vi "HFRR ADV v015 new software.vi"() -> ()   [LabVIEW 2025] (continued)
        n324 = event-data() -> ()  [unwired: 1 in, 6 out]
        n325 = Unbundle By Name("Password 3") -> ("Service Password"=w414:string)
        n326 = call <vilib>:"Trim Whitespace.vi"("string"=w414) -> ("trimmed string"=w412:string)  [unwired: 1 in]
        n327 = Equal?(x=w412, y="Service@123") -> (x = y?=w413:bool)
        n328 = case shown="False" w413 {
          selector: w413 -> [w418 w420]
          frame False {
            n329 = local write "Service Password enable"(w418) -> ()
            n330 = property on="Service Password Log" class="Str"("Visible"=TRUE) -> ()  [unwired: 2 in, 2 out]
            n331 = property on="Tab Control 5" class="TabCtl (strict)"("Tabs Visible?"=TRUE ("Page Labels Display Visible?")) -> ()  [unwired: 2 in, 2 out]
          }
          frame True {
            n332 = property on="Service Password Log" class="Str"("Visible"=FALSE) -> ()  [unwired: 2 in, 2 out]
            "Service Password enable" <- w420
          }
        }
      }
      event "Sign In": Value Change {
        w422 = FALSE ("Visible")
        n333 = event-data() -> ()  [unwired: 1 in, 6 out]
        n334 = property on="About" class="Clust (strict)"("Visible"=w422) -> ()  [unwired: 2 in, 2 out]
        n335 = property on="Password 3" class="Clust (strict)"("Visible"=w422) -> ()  [unwired: 2 in, 2 out]
        n336 = property on="Service Password Log" class="Str"("Visible"=FALSE) -> ()  [unwired: 2 in, 2 out]
      }
      event "Info": Value Change {
        n337 = event-data() -> ()  [unwired: 1 in, 6 out]
        n338 = local read "Info"() -> (w424:bool)
        n339 = case shown="False" w424 {
          frame False {
            n340 = property on="About" class="Clust (strict)"("Visible"=FALSE) -> ()  [unwired: 2 in, 2 out]
          }
          frame True {
            n341 = property on="About" class="Clust (strict)"("Visible"=TRUE) -> ()  [unwired: 2 in, 2 out]
          }
        }
      }
      event "Calibration": Value Change {
        n342 = event-data() -> ()  [unwired: 1 in, 6 out]
        n343 = local read "Calibration"() -> (w428:bool)
        n344 = case shown="False" w428 {
          frame False {
            n345 = property on="Calibration 2" class="TabCtl (strict)"("Visible"=FALSE) -> ()  [unwired: 2 in, 2 out]
            n346 = local write "Cal Password"("" ("Cal Password")) -> ()
          }
          frame True {
            n347 = property on="Calibration 2" class="TabCtl (strict)"("Visible"=TRUE) -> ()  [unwired: 2 in, 2 out]
            n348 = local write "Cal Password"("" ("Cal Password")) -> ()
          }
        }
        n349 = property on="Wrong Password" class="Str"("Visible"=FALSE) -> ()  [unwired: 2 in, 2 out]
      }
      event "Cal Password": Value Change {
        n350 = event-data() -> ()  [unwired: 1 in, 6 out]
        n351 = local read "Cal Password"() -> (w436:string)
        n352 = call <vilib>:"Trim Whitespace.vi"("string"=w436) -> ("trimmed string"=w435:string)  [unwired: 1 in]
        n353 = Equal?(x=w435, y="Cal@321") -> (x = y?=w433:bool)
        n354 = case shown="True" w433 {
          frame False {
            n355 = property on="Wrong Password" class="Str"("Visible"=TRUE) -> ()  [unwired: 2 in, 2 out]
          }
          frame True {
            n356 = property on="Wrong Password" class="Str"("Visible"=FALSE) -> ()  [unwired: 2 in, 2 out]
            n357 = local write "Main Tab"(T2."About" ("Main Tab")) -> ()
            n358 = local write "Cal Password"("" ("Cal Password")) -> ()
            n359 = local write "Main Dashboard Buttons"(T1."About" ("Main Dashboard Buttons")) -> ()
            n360 = local write "Tab Control 5"(T12."Temperature Calibration" ("Tab Control 5")) -> ()
            n361 = property on="Calibration 2" class="TabCtl (strict)"("Visible"=FALSE) -> ()  [unwired: 2 in, 2 out]
            n362 = property on="Tab Control 5" class="TabCtl (strict)"("Tabs Visible?"=FALSE ("Page Labels Display Visible?")) -> ()  [unwired: 2 in, 2 out]
            n363 = local write "Calibration"(FALSE ("Calibration")) -> ()
          }
        }
      }
      event "Calibration Selection": Value Change {
        n364 = event-data() -> ()  [unwired: 1 in, 6 out]
        n365 = local read "Calibration Selection"() -> (w447:T8)
        n366 = case shown="\"Stroke Calibration\"" w447 {
          tunnel: [T7."Stroke" ("Main Calibration Tab") T7."Friction" ("Main Calibration Tab") T7."Main" ("Main Calibration Tab") T7."Temperature" ("Main Calibration Tab")] -> w446
          frame "Stroke Calibration" {
          }
          frame "Friction Force Calibration" {
          }
          frame Default {
          }
          frame "Temperature Calibration" {
          }
        }
        n367 = local write "Main Calibration Tab"(w446) -> ()
      }
      event "Back Stroke": Value Change {
        n368 = event-data() -> ()  [unwired: 1 in, 6 out]
        n369 = local write "Main Stroke Tab"(T9."Step 1" ("Main Stroke Tab")) -> ()
        n370 = local write "Main Calibration Tab"(T7."Main" ("Main Calibration Tab")) -> ()
        n371 = local write "Back Stroke"(FALSE ("Back Stroke")) -> ()
      }
      event "Step 2 Back": Value Change {
        n372 = event-data() -> ()  [unwired: 1 in, 6 out]
        n373 = local write "Main Stroke Tab"(T9."Step 1" ("Main Stroke Tab")) -> ()
        n374 = local write "Step 2 Back"(FALSE ("Back Stroke")) -> ()
      }
      event "Step 3 Back": Value Change {
        n375 = event-data() -> ()  [unwired: 1 in, 6 out]
        n376 = local write "Main Stroke Tab"(T9."Step 2" ("Main Stroke Tab")) -> ()
        n377 = local write "Step 3 Back"(FALSE ("Back Stroke")) -> ()
      }
      event "Step 4 Back": Value Change {
        n378 = event-data() -> ()  [unwired: 1 in, 6 out]
        n379 = local write "Main Stroke Tab"(T9."Step 3" ("Main Stroke Tab")) -> ()
        n380 = local write "Step 4 Back"(FALSE ("Back Stroke")) -> ()
      }
      event "Step 5 Back": Value Change {
        n381 = event-data() -> ()  [unwired: 1 in, 6 out]
        n382 = local write "Main Stroke Tab"(T9."Step 4" ("Main Stroke Tab")) -> ()
        n383 = local write "Step 5 Back"(FALSE ("Back Stroke")) -> ()
      }
      event "Step 6 Back": Value Change {
        n384 = event-data() -> ()  [unwired: 1 in, 6 out]
        n385 = local write "Main Stroke Tab"(T9."Step 5" ("Main Stroke Tab")) -> ()
        n386 = local write "Step 6 Back"(FALSE ("Back Stroke")) -> ()
      }
      event "Back Stroke step 7": Value Change {
        n387 = event-data() -> ()  [unwired: 1 in, 6 out]
        n388 = local write "Main Stroke Tab"(T9."Step 6" ("Main Stroke Tab")) -> ()
        n389 = local write "Back Stroke step 7"(FALSE ("Back Stroke")) -> ()
      }
      event "Back Stroke step 8": Value Change {
        n390 = event-data() -> ()  [unwired: 1 in, 6 out]
        n391 = local write "Main Stroke Tab"(T9."Step 7" ("Main Stroke Tab")) -> ()
        n392 = local write "Back Stroke step 8"(FALSE ("Back Stroke")) -> ()
      }
      event "Back Stroke 8": Value Change {
        n393 = event-data() -> ()  [unwired: 1 in, 6 out]
        n394 = local write "MOVE CARRIAGE TO"(0.0 ("MOVE CARRIAGE TO")) -> ()
        n395 = local write "Main Stroke Tab"(T9."Step 1" ("Main Stroke Tab")) -> ()
        n396 = local write "Back Stroke 8"(FALSE ("Back Stroke 8")) -> ()
      }
      event "Continue Stroke": Value Change {
        n397 = event-data() -> ()  [unwired: 1 in, 6 out]
        n398 = local write "Main Stroke Tab"(T9."Step 2" ("Main Stroke Tab")) -> ()
        n399 = local write "Continue Stroke"(FALSE ("Continue Stroke")) -> ()
      }
      event "Continue Stroke step 2": Value Change {
        n400 = event-data() -> ()  [unwired: 1 in, 6 out]
        n401 = local write "Main Stroke Tab"(T9."Step 3" ("Main Stroke Tab")) -> ()
        n402 = local write "Continue Stroke step 2"(FALSE ("Continue Stroke")) -> ()
      }
      event "Continue Stroke step 3": Value Change {
        n403 = event-data() -> ()  [unwired: 1 in, 6 out]
        n404 = local write "Main Stroke Tab"(T9."Step 4" ("Main Stroke Tab")) -> ()
        n405 = local write "Continue Stroke step 3"(FALSE ("Continue Stroke")) -> ()
      }
      event "Continue Stroke step 4": Value Change {
        n406 = event-data() -> ()  [unwired: 1 in, 6 out]
        n407 = local write "Main Stroke Tab"(T9."Step 5" ("Main Stroke Tab")) -> ()
        n408 = local write "Continue Stroke step 4"(FALSE ("Continue Stroke")) -> ()
      }
      event "Continue Stroke step 5": Value Change {
        n409 = event-data() -> ()  [unwired: 1 in, 6 out]
        n410 = local write "Main Stroke Tab"(T9."Step 6" ("Main Stroke Tab")) -> ()
        n411 = local write "Continue Stroke step 5"(FALSE ("Continue Stroke")) -> ()
      }
      event "Continue Stroke step 6": Value Change {
        n412 = event-data() -> ()  [unwired: 1 in, 6 out]
        n413 = local write "Main Stroke Tab"(T9."Step 7" ("Main Stroke Tab")) -> ()
        n414 = local write "Continue Stroke step 6"(FALSE ("Continue Stroke")) -> ()
      }
      event "Continue Stroke step 7": Value Change {
        w485 = FALSE ("0.2mm")
        n415 = event-data() -> ()  [unwired: 1 in, 6 out]
        n416 = local write "0.4 mm"(w485) -> ()
        n417 = local write "0.6 mm"(w485) -> ()
        n418 = local write "1.0 mm"(w485) -> ()
        n419 = local write "1.2 mm"(w485) -> ()
        n420 = local write "0.2 2"(w485) -> ()
        n421 = local write "0.4 2"(w485) -> ()
        n422 = local write "0.6 2"(w485) -> ()
        n423 = local write "0.8 2"(w485) -> ()
        n424 = local write "1.0 2"(w485) -> ()
        n425 = local write "1.2"(w485) -> ()
        n426 = local write "0.2mm"(w485) -> ()
        n427 = local write "0.8mm"(w485) -> ()
        n428 = local write "Main Stroke Tab"(T9."Step 8" ("Main Stroke Tab")) -> ()
        n429 = local write "Continue Stroke step 7"(FALSE ("Continue Stroke")) -> ()
        n430 = local write "Stroke Test Complete"(T10."Test Progress" ("Stroke Test Complete")) -> ()
        "Position Measurment Temp" <- 0.0 ("Position Measurment Temp")
        "Calibration Tare" <- TRUE ("Calibration Tare")
      }
      event "Continue Stroke step 8": Value Change {
        n431 = event-data() -> ()  [unwired: 1 in, 6 out]
        n432 = local read "LVDT STROKE  Calibration"() -> (w490:dbl)
        n433 = local read "Position Measurment Temp"() -> (w491:dbl)
        n434 = case shown="7" w491 {
          selector: w491 -> [w496 w501 w506 w511 w516 w521 w524 w525]
          tunnel: w490 -> [w492 w497 w502 w507 w512 w517 _ _]
          frame 0, Default {
            w494 = TRUE ("0.2mm")
            n435 = Increment(x=w496) -> (x+1=w495:i32)
            n436 = local write "Position Measurment Temp"(w495) -> ()
            n437 = local write "0.2mm"(w494) -> ()
            n438 = local write "0.2 2"(w494) -> ()
            n439 = local write "MOVE CARRIAGE TO"(0.2 ("MOVE CARRIAGE TO")) -> ()
            "Calibration 0.2" <- w492
          }
          frame 1 {
            w499 = TRUE ("0.4 mm")
            n440 = Increment(x=w501) -> (x+1=w500:i32)
            n441 = local write "Calibration 0.4"(w497) -> ()
            n442 = local write "Position Measurment Temp"(w500) -> ()
            n443 = local write "0.4 mm"(w499) -> ()
            n444 = local write "MOVE CARRIAGE TO"(0.4 ("MOVE CARRIAGE TO")) -> ()
            n445 = local write "0.4 2"(w499) -> ()
          }
          frame 2 {
            w504 = TRUE ("0.6 mm")
            n446 = Increment(x=w506) -> (x+1=w505:i32)
            n447 = local write "Calibration 0.6"(w502) -> ()
            n448 = local write "Position Measurment Temp"(w505) -> ()
            n449 = local write "0.6 2"(w504) -> ()
            n450 = local write "0.6 mm"(w504) -> ()
            n451 = local write "MOVE CARRIAGE TO"(0.6 ("MOVE CARRIAGE TO")) -> ()
          }
          frame 3 {
            w508 = TRUE ("0.6 mm")
            n452 = Increment(x=w511) -> (x+1=w510:i32)
            n453 = local write "Position Measurment Temp"(w510) -> ()
            n454 = local write "MOVE CARRIAGE TO"(0.8 ("MOVE CARRIAGE TO")) -> ()
            n455 = local write "0.8mm"(w508) -> ()
            n456 = local write "0.8 2"(w508) -> ()
            "Calibration 0.8" <- w507
          }
          frame 4 {
            w513 = TRUE ("0.6 mm")
            n457 = Increment(x=w516) -> (x+1=w515:i32)
            n458 = local write "Position Measurment Temp"(w515) -> ()
            n459 = local write "MOVE CARRIAGE TO"(1.0 ("MOVE CARRIAGE TO")) -> ()
            n460 = local write "1.0 mm"(w513) -> ()
            n461 = local write "1.0 2"(w513) -> ()
            "Calibration 1.0" <- w512
          }
          frame 5 {
            w518 = TRUE ("0.6 mm")
            n462 = Increment(x=w521) -> (x+1=w520:i32)
            n463 = local write "Position Measurment Temp"(w520) -> ()
            n464 = local write "MOVE CARRIAGE TO"(1.2 ("MOVE CARRIAGE TO")) -> ()
            n465 = local write "1.2 mm"(w518) -> ()
            n466 = local write "1.2"(w518) -> ()
            "Calibration 1.2" <- w517
          }
          frame 6 {
            n467 = Increment(x=w524) -> (x+1=w523:i32)
            n468 = local write "Position Measurment Temp"(w523) -> ()
            n469 = local write "Stroke Test Complete"(T10."Stroke Points Completed" ("Stroke Test Complete")) -> ()
          }
          frame 7 {
            n470 = stacked-sequence {
              tunnel: w525 -> [w526 _ _]
              frame #0 {
                n471 = Increment(x=w526) -> (x+1=w527:i32)
                n472 = local write "Main Stroke Tab"(T9."Step 9" ("Main Stroke Tab")) -> ()
                n473 = local write "Position Measurment Temp"(w527) -> ()
                n474 = Insert Into Array(array=dbl[] [], new element #1=0.2 ("new element/subarray"), new element #2=0.4 ("new element/subarray"), new element #3=0.6 ("new element/subarray"), new element #4=0.8 ("new element/subarray"), new element #5=1.0 ("new element/subarray"), new element #6=1.2 ("new element/subarray")) -> (→"1D stroke":dbl[])  [unwired: 1 in]
                n475 = local read "Calibration 0.2"() -> (w534:dbl)
                n476 = local read "Calibration 0.4"() -> (w533:dbl)
                n477 = local read "Calibration 0.6"() -> (w532:dbl)
                n478 = local read "Calibration 0.8"() -> (w531:dbl)
                n479 = local read "Calibration 1.0"() -> (w530:dbl)
                n480 = local read "Calibration 1.2"() -> (w529:dbl)
                n481 = Insert Into Array(array=dbl[] [], new element #1=w534, new element #2=w533, new element #3=w532, new element #4=w531, new element #5=w530, new element #6=w529) -> (→"Calibrated Voltage Value":dbl[])  [unwired: 1 in]
              }
              frame #1 {
                n482 = local read "Calibrated Voltage Value"() -> (w546:dbl[])
                n483 = local read "1D stroke"() -> (w547:dbl[])
                n484 = for {
                  tunnel: [w550] -> w545 mode=indexing
                  tunnel: w547 -> [w549] mode=indexing
                  tunnel: w546 -> [w548] mode=indexing
                  n485 = formula code="if (stroke == 0.2) {\n    status = (voltage >= 0.0961 && voltage <= 0.4961) ? 1 : 0;\n} else if (stroke == 0.4) {\n    status = (voltage >= 0.3425 && voltage <= 0.7425) ? 1 : 0;\n} else if (stroke == 0.6) {\n    status = (voltage >= 0.5370 && voltage <= 0.9370) ? 1 : 0;\n} else if (stroke == 0.8) {\n    status = (voltage >= 0.6640 && voltage <= 1.0640) ? 1 : 0;\n} else if (stroke == 1.0) {\n    status = (voltage >= 0.9000 && voltage <= 1.1000) ? 1 : 0;\n} else if (stroke == 1.2) {\n    status = (voltage >= 0.9278 && voltage <= 1.3278) ? 1 : 0;\n} else {\n    status = 0; // Fails if an invalid stroke value is supplied\n}"("stroke"=w549, "voltage"=w548) -> ("status"=w550:dbl)
                }
                "Status" <- w545
              }
              frame #2 {
                w557 = 1.0
                n486 = local read "Status"() -> (w564:dbl[])
                n487 = Index Array(array=w564) -> (element #1=w563:dbl, element #2=w562:dbl, element #3=w561:dbl, element #4=w560:dbl, element #5=w559:dbl, element #6=w558:dbl)  [unwired: 6 in]
                n488 = Equal?(x=w562, y=w557) -> (x = y?=w555:bool)
                n489 = Equal?(x=w561, y=w557) -> (x = y?=w554:bool)
                n490 = Equal?(x=w560, y=w557) -> (x = y?=w553:bool)
                n491 = Equal?(x=w559, y=w557) -> (x = y?=w552:bool)
                n492 = Equal?(x=w558, y=w557) -> (x = y?=w551:bool)
                n493 = Equal?(x=w563, y=w557) -> (x = y?=w556:bool)
                n494 = case shown="True" w556 {
                  selector: w556 -> [w575 w576]
                  frame True {
                    n495 = local write "Point 1 - 0.2 mm"(w575) -> ()
                    n496 = property on="Point 1 - 0.2 mm" class="Bool"("Caption.Visible"=w575) -> ()  [unwired: 2 in, 2 out]
                  }
                  frame False {
                    n497 = local write "Point 1 - 0.2 mm"(w576) -> ()
                    n498 = property on="Point 1 - 0.2 mm" class="Bool"("Caption.Visible"=w576) -> ()  [unwired: 2 in, 2 out]
                  }
                }
                n499 = case shown="True" w555 {
                  selector: w555 -> [w573 w574]
                  frame True {
                    n500 = local write "Point 2 - 0.4 mm"(w573) -> ()
                    n501 = property on="Point 2 - 0.4 mm" class="Bool"("Caption.Visible"=w573) -> ()  [unwired: 2 in, 2 out]
                  }
                  frame False {
                    n502 = local write "Point 2 - 0.4 mm"(w574) -> ()
                    n503 = property on="Point 2 - 0.4 mm" class="Bool"("Caption.Visible"=w574) -> ()  [unwired: 2 in, 2 out]
                  }
                }
                n504 = case shown="True" w552 {
                  selector: w552 -> [w567 w568]
                  frame True {
                    n505 = local write "Point 5 - 1.0 mm"(w567) -> ()
                    n506 = property on="Point 5 - 1.0 mm" class="Bool"("Caption.Visible"=w567) -> ()  [unwired: 2 in, 2 out]
                  }
                  frame False {
                    n507 = local write "Point 5 - 1.0 mm"(w568) -> ()
                    n508 = property on="Point 5 - 1.0 mm" class="Bool"("Caption.Visible"=w568) -> ()  [unwired: 2 in, 2 out]
                  }
                }
                n509 = case shown="True" w554 {
                  selector: w554 -> [w571 w572]
                  frame True {
                    n510 = local write "Point 3 - 0.6 mm"(w571) -> ()
                    n511 = property on="Point 3 - 0.6 mm" class="Bool"("Caption.Visible"=w571) -> ()  [unwired: 2 in, 2 out]
                  }
                  frame False {
                    n512 = local write "Point 3 - 0.6 mm"(w572) -> ()
                    n513 = property on="Point 3 - 0.6 mm" class="Bool"("Caption.Visible"=w572) -> ()  [unwired: 2 in, 2 out]
                  }
                }
                n514 = case shown="True" w553 {
                  selector: w553 -> [w569 w570]
                  frame True {
                    n515 = local write "Point 4 - 0.8 mm"(w569) -> ()
                    n516 = property on="Point 4 - 0.8 mm" class="Bool"("Caption.Visible"=w569) -> ()  [unwired: 2 in, 2 out]
                  }
                  frame False {
                    n517 = local write "Point 4 - 0.8 mm"(w570) -> ()
                    n518 = property on="Point 4 - 0.8 mm" class="Bool"("Caption.Visible"=w570) -> ()  [unwired: 2 in, 2 out]
                  }
                }
                n519 = case shown="True" w551 {
                  selector: w551 -> [w565 w566]
                  frame True {
                    n520 = local write "Point 6 - 1.2 mm"(w565) -> ()
                    n521 = property on="Point 6 - 1.2 mm" class="Bool"("Caption.Visible"=w565) -> ()  [unwired: 2 in, 2 out]
                  }
                  frame False {
                    n522 = local write "Point 6 - 1.2 mm"(w566) -> ()
                    n523 = property on="Point 6 - 1.2 mm" class="Bool"("Caption.Visible"=w566) -> ()  [unwired: 2 in, 2 out]
                  }
                }
              }
            }
          }
        }
      }
      event "TEMPERATURE STEP Back 1", "TEMPERATURE STEP Back air Temp": Value Change {
        n524 = event-data() -> ()  [unwired: 1 in, 6 out]
        n525 = stacked-sequence {
          frame #0 {
            n526 = local write "Main Calibration Tab"(T7."Main" ("Main Calibration Tab")) -> ()
          }
          frame #1 {
            n527 = Wait (ms)(milliseconds to wait=u32 1000) -> ()  [unwired: 1 out]
          }
          frame #2 {
            n528 = local write "Command"("CAL;END" ("Command")) -> ()
          }
          frame #3 {
            n529 = Wait (ms)(milliseconds to wait=u32 2000) -> ()  [unwired: 1 out]
          }
          frame #4 {
            n530 = local write "Command"("CAL;END" ("Command")) -> ()
          }
        }
      }
      event "Temperature Continue Step 1": Value Change {
        n531 = event-data() -> ()  [unwired: 1 in, 6 out]
        n532 = stacked-sequence {
          frame #0 {
            n533 = Wait (ms)(milliseconds to wait=u32 1500) -> ()  [unwired: 1 out]
          }
          frame #1 {
            n534 = local write "Command"("CAL;START" ("Command")) -> ()
          }
          frame #2 {
            n535 = local write "Tab Control 4"(T11."Step 2" ("Tab Control 4")) -> ()
            n536 = Wait (ms)(milliseconds to wait=u32 1500) -> ()  [unwired: 1 out]
          }
          frame #3 {
            n537 = local write "Command"("CAL;START" ("Command")) -> ()
          }
          frame #4 {
            n538 = Wait (ms)(milliseconds to wait=u32 2000) -> ()  [unwired: 1 out]
          }
          frame #5 {
            # "CAL;A1;<true_T>"
            n539 = local write "Command"("CAL;A1;0" ("Command")) -> ()
          }
          frame #6 {
            n540 = Wait (ms)(milliseconds to wait=u32 2000) -> ()  [unwired: 1 out]
          }
          frame #7 {
            # "CAL;A1;<true_T>"
            n541 = local write "Command"("CAL;A1;0" ("Command")) -> ()
          }
        }
      }
      event "Temperature Continue Step air Step 1": Value Change {
        n542 = event-data() -> ()  [unwired: 1 in, 6 out]
        n543 = stacked-sequence {
          frame #0 {
            n544 = Wait (ms)(milliseconds to wait=u32 1500) -> ()  [unwired: 1 out]
          }
          frame #1 {
            n545 = local write "Command"("CAL;START" ("Command")) -> ()
          }
          frame #2 {
            n546 = local write "Tab Control 4"(T11."Air Step 2" ("Tab Control 4")) -> ()
            n547 = Wait (ms)(milliseconds to wait=u32 1500) -> ()  [unwired: 1 out]
          }
          frame #3 {
            n548 = local write "Command"("CAL;START" ("Command")) -> ()
          }
          frame #4 {
            n549 = Wait (ms)(milliseconds to wait=u32 2000) -> ()  [unwired: 1 out]
          }
          frame #5 {
            # "CAL;A1;<true_T>"
            n550 = local write "Command"("CAL;A2;0" ("Command")) -> ()
          }
          frame #6 {
            n551 = Wait (ms)(milliseconds to wait=u32 2000) -> ()  [unwired: 1 out]
          }
          frame #7 {
            # "CAL;A1;<true_T>"
            n552 = local write "Command"("CAL;A1;0" ("Command")) -> ()
          }
        }
      }
      event "Quit": Value Change {
        n553 = event-data() -> ()  [unwired: 1 in, 6 out]
      }
    }
    n554 = Wait (ms)(milliseconds to wait=u32 100) -> ()  [unwired: 1 out]
  }
  n555 = while {
    stop <- w602 stop-if-true
    n556 = Wait (ms)(milliseconds to wait=u32 200) -> ()  [unwired: 1 out]
    n557 = local read "Quit"() -> (w602:bool)
  }
  n558 = while {
    shift-right: [w604] -> _
    shift-left: "Enum - Selector" -> [w605]
    stop <- w606 stop-if-true
    # "Auto Start Logic Loop"
    n559 = case shown="\"Maintain Stage\"" w605 {
      tunnel: [w609 w615 w642 w674 w704 Auto_Start_enum."Exit" ("Enum - Selector") Auto_Start_enum."Init" ("Enum - Selector")] -> w604
      frame "Init", Default {
        n560 = local read "Auto Start Test"() -> (w608:bool)
        n561 = Select(t=Auto_Start_enum."Humidity & Temperature On" ("Enum - Selector"), s=w608, f=Auto_Start_enum."Init") -> (s? t:f=w609:T15)
      }
      frame "Humidity & Temperature On" {
        n562 = stacked-sequence {
          tunnel: [_ _ _ _ _ _ Auto_Start_enum."Reach point" ("Enum - Selector")] -> w612
          frame #0 {
            w617 = T18."Disabled and Grayed Out" ("Disabled")
            w618 = TRUE ("Heater Button")
            n563 = property on="Humidity" class="Bool (strict)"("DisabledEnum"=w617) -> ()  [unwired: 2 in, 2 out]
            n564 = property on="Heater Button" class="Bool (strict)"("DisabledEnum"=w617) -> ()  [unwired: 2 in, 2 out]
            n565 = local write "Heater Button"(w618) -> ()
            n566 = local write "Humidity"(w618) -> ()
            n567 = property on="Heater Button" class="Bool (strict)"("Val(Sgnl)"=TRUE ("Value (Signaling)")) -> ()  [unwired: 2 in, 2 out]
          }
          frame #1 {
            n568 = Wait (ms)(milliseconds to wait=u32 3000) -> ()  [unwired: 1 out]
          }
          frame #2 {
            n569 = local read "Set Temp"() -> (w624:dbl)
            n570 = Number To Fractional String(number=w624, precision (6)=i16 2) -> (F-format string=w621:string)  [unwired: 2 in]
            n571 = Concatenate Strings("ST;" ("Command"), w621) -> (w622:string)
            n572 = local write "Command"(w622) -> ()
          }
          frame #3 {
            n573 = Wait (ms)(milliseconds to wait=u32 1500) -> ()  [unwired: 1 out]
          }
          frame #4 {
            (unwired) i16 2 ("precision (6)")
            n574 = local read "Set Rh"() -> (w627:dbl)
            n575 = Number To Fractional String(number=w627) -> (F-format string=w630:string)  [unwired: 3 in]
            n576 = local read "WriteHumidity"() -> (w628:string[])
            n577 = Concatenate Strings("M;" ("new element/subarray"), w630) -> (w631:string)
            n578 = local write "Command"("HE;1" ("Command")) -> ()
            n579 = Insert Into Array(array=w628, new element=w631) -> (w629:string[])  [unwired: 1 in]
            n580 = local write "WriteHumidity"(w629) -> ()
          }
          frame #5 {
            n581 = Wait (ms)(milliseconds to wait=u32 1500) -> ()  [unwired: 1 out]
          }
          frame #6 {
            w634 = TRUE ("Reach point temp")
            n582 = local write "Reach point Humidity"(w634) -> ()
            n583 = local write "Reach point temp"(w634) -> ()
          }
        }
        n584 = local read "Auto Start Test"() -> (w614:bool)
        n585 = Not(x=w614) -> (.not. x?=w613:bool)
        n586 = Select(t=Auto_Start_enum."close", s=w613, f=w612) -> (s? t:f=w615:T15)
      }
      frame "Reach point" {
        w643 = TRUE ("PAUSE")
        w651 = 1.0 ("y")
        w654 = 1.0 ("y")
        n587 = local read "Set Temp"() -> (w636:dbl)
        n588 = local read "Set Humidity:"() -> (w650:dbl)
        n589 = local read "Humidity ( %RH )"() -> (w655:dbl)
        n590 = Add(x=w636, y=w654) -> (x+y=w653:dbl)
        n591 = Subtract(x=w636, y=w654) -> (x-y=w652:dbl)
        n592 = Add(x=w650, y=w651) -> (x+y=w649:dbl)
        n593 = Subtract(x=w650, y=w651) -> (x-y=w648:dbl)
        n594 = local read "TEMP"() -> (w656:dbl)
        n595 = In Range and Coerce(upper limit=w649, x=w655, lower limit=w648) -> (In Range?=w637:bool)  [unwired: 1 out]
        n596 = In Range and Coerce(upper limit=w653, x=w656, lower limit=w652) -> (In Range?=w638:bool)  [unwired: 1 out]
        n597 = case shown="True" w637 {
          frame False {
          }
          frame True {
            n598 = case shown="True" "Reach point Humidity" {
              selector: "Reach point Humidity" -> [_ w662]
              frame False {
              }
              frame True {
                n599 = local read "EVENT LOG"() -> (w659:string)
                n600 = Not(x=w662) -> (.not. x?=w661:bool)
                n601 = local write "Reach point Humidity"(w661) -> ()
                n602 = call "Event Log.vi"("Content"="Target Humidity reached", "EVENT LOG"=w659) -> ("EVENT LOG"=w660:string)  [unwired: 8 in, 1 out]
                n603 = local write "EVENT LOG"(w660) -> ()
              }
            }
          }
        }
        n604 = case shown="True" w638 {
          frame False {
          }
          frame True {
            n605 = case shown="True" "Reach point temp" {
              selector: "Reach point temp" -> [_ w668]
              frame False {
              }
              frame True {
                n606 = local read "EVENT LOG"() -> (w665:string)
                n607 = Not(x=w668) -> (.not. x?=w667:bool)
                n608 = local write "Reach point temp"(w667) -> ()
                n609 = call "Event Log.vi"("Content"="Target Temperature reached", "EVENT LOG"=w665) -> ("EVENT LOG"=w666:string)  [unwired: 8 in, 1 out]
                n610 = local write "EVENT LOG"(w666) -> ()
              }
            }
          }
        }
        n611 = local read "Auto Start Test"() -> (w641:bool)
        n612 = And(x=w638, y=w637) -> (x .and. y?=w647:bool)
        n613 = Select(t=Auto_Start_enum."Maintain Stage" ("Enum - Selector"), s=w647, f=Auto_Start_enum."Reach point" ("Enum - Selector")) -> (s? t:f=w644:T15)
        n614 = Not(x=w641) -> (.not. x?=w640:bool)
        n615 = Select(t=Auto_Start_enum."close", s=w640, f=w644) -> (s? t:f=w642:T15)
        n616 = call "ELAPSED TIMER VI.vi"("RESET"=w643, "PAUSE"=w643) -> ()  [unwired: 7 in, 3 out]
      }
      frame "Maintain Stage" {
        w683 = 2.0 ("y")
        w682 = 1.0 ("y")
        # "Humidity and  temperatures Set Point  have been reached"
        n617 = local read "Set Temp"() -> (w669:dbl)
        n618 = local read "Set Humidity:"() -> (w686:dbl)
        n619 = local read "Humidity ( %RH )"() -> (w689:dbl)
        n620 = Add(x=w669, y=w682) -> (x+y=w688:dbl)
        n621 = Subtract(x=w669, y=w682) -> (x-y=w687:dbl)
        n622 = local read "TEMP"() -> (w690:dbl)
        n623 = Add(x=w686, y=w683) -> (x+y=w685:dbl)
        n624 = Subtract(x=w686, y=w683) -> (x-y=w684:dbl)
        n625 = In Range and Coerce(upper limit=w688, x=w690, lower limit=w687) -> (In Range?=w681:bool)  [unwired: 1 out]
        n626 = In Range and Coerce(upper limit=w685, x=w689, lower limit=w684) -> (In Range?=w680:bool)  [unwired: 1 out]
        n627 = And(x=w681, y=w680) -> (x .and. y?=w679:bool)
        n628 = Not(x=w679) -> (.not. x?=w678:bool)
        n629 = call "ELAPSED TIMER VI.vi"("TARGET"=60.0, "RESET"=w678, "PAUSE"=FALSE) -> ("ELAPSED INDICATION"=w675:bool)  [unwired: 6 in, 2 out]
        n630 = case shown="True" w675 {
          tunnel: w675 -> [_ w693]
          tunnel: [Auto_Start_enum."Maintain Stage" ("Enum - Selector") w692] -> w673
          frame False {
          }
          frame True {
            n631 = stacked-sequence {
              tunnel: w693 -> [_ _ _ _ _]
              tunnel: [_ _ _ _ Auto_Start_enum."Start Stage" ("Enum - Selector")] -> w692
              frame #0 {
                n632 = local read "EVENT LOG"() -> (w695:string)
                n633 = call "Event Log.vi"("Content"="Humidity and temperature set point has stabilized.", "EVENT LOG"=w695) -> ("EVENT LOG"=w696:string)  [unwired: 8 in, 1 out]
                n634 = local write "EVENT LOG"(w696) -> ()
              }
              frame #1 {
                n635 = Wait (ms)(milliseconds to wait=u32 100) -> ()  [unwired: 1 out]
              }
              frame #2 {
                n636 = local read "EVENT LOG"() -> (w699:string)
                n637 = call "Event Log.vi"("Content"="Auto Test Started", "EVENT LOG"=w699) -> ("EVENT LOG"=w700:string)  [unwired: 8 in, 1 out]
                n638 = local write "EVENT LOG"(w700) -> ()
              }
              frame #3 {
                w701 = TRUE ("RUN")
                n639 = local write "RUN"(w701) -> ()
                n640 = property on="Auto Start Temp" class="Bool (strict)"("Val(Sgnl)"=w701) -> ()  [unwired: 2 in, 2 out]
                "Auto Start Temp" <- w701
              }
              frame #4 {
              }
            }
          }
        }
        n641 = local read "Auto Start Test"() -> (w672:bool)
        n642 = Not(x=w672) -> (.not. x?=w671:bool)
        n643 = Select(t=Auto_Start_enum."close", s=w671, f=w673) -> (s? t:f=w674:T15)
      }
      frame "Start Stage" {
        w703 = TRUE ("PAUSE")
        n644 = local read "Auto Start Test"() -> (w708:bool)
        n645 = Not(x=w708) -> (.not. x?=w707:bool)
        n646 = Select(t=Auto_Start_enum."close" ("Enum - Selector"), s=w707, f=Auto_Start_enum."Start Stage" ("Enum - Selector")) -> (s? t:f=w704:T15)
        n647 = call "ELAPSED TIMER VI.vi"("RESET"=w703, "PAUSE"=w703) -> ()  [unwired: 7 in, 3 out]
      }
      frame "close" {
        w710 = FALSE ("Heater Button")
        n648 = local write "RUN"(w710) -> ()
        n649 = local write "Heater Button"(w710) -> ()
        n650 = local write "Humidity"(w710) -> ()
        n651 = local write "Auto Start Test"(w710) -> ()
        n652 = property on="Heater Button" class="Bool (strict)"("Val(Sgnl)"=FALSE ("Value (Signaling)")) -> ()  [unwired: 2 in, 2 out]
      }
      frame "Exit" {
      }
    }
    n653 = Wait (ms)(milliseconds to wait=u32 100) -> ()  [unwired: 1 out]
    n654 = local read "Quit"() -> (w606:bool)
  }
  n655 = property on="Service Password Log" class="Str"("Visible"=w14) -> ()  [unwired: 2 in, 2 out]
  n656 = property on="Password 3" class="Clust (strict)"("Visible"=w14) -> ()  [unwired: 2 in, 2 out]
  n657 = while {
    stop <- w739 stop-if-true
    w722 = errorcluster {"status"=FALSE, "code"=0, "source"=""} ("error in (no error) 3")
    # "this loop is for manual report generation"
    n658 = local read "Confirm Measrurement"() -> (w721:bool)
    n659 = case shown="True" w721 {
      selector: w721 -> [_ w829]
      tunnel: errorcluster {"status"=FALSE, "code"=0, "source"=""} ("error in (no error) 3") -> [_ w830]
      tunnel: [_ w828] -> _
      frame False {
      }
      frame True {
        n660 = stacked-sequence {
          tunnel: w830 -> [_ w863 _]
          tunnel: w829 -> [_ _ w970]
          tunnel: [_ w851 _] -> w828
          frame #0 {
            n661 = String To Path(string="C:\\LAB-IQ\\Image Calibrate v01.dcf") -> (path=w833:path)
            n662 = Open/Create/Replace File ("Open File")(file path (use dialog)=w833) -> (refnum out=w834:refnum<file>)  [unwired: 5 in, 2 out]
            n663 = for {
              N: 4 -> [_]
              tunnel: w834 -> [w840]
              i -> [w836]
              n664 = Read from Text File ("Read File")(file (use dialog)=w840) -> (text=w841:string)  [unwired: 3 in, 3 out]
              n665 = String Subset(string=w841, offset (0)=6, length (rest)=10 ("length (rest)")) -> (substring=w837:string)
              n666 = Fract/Exp String To Number(string=w837) -> (number=w835:dbl)  [unwired: 3 in, 1 out]
              n667 = case shown="3" w836 {
                tunnel: w835 -> [w842 w843 _ w844 _]
                frame 0 {
                  n668 = local write "5x Gain"(w842) -> ()
                }
                frame 1 {
                  n669 = local write "10x Gain"(w843) -> ()
                }
                frame 2 {
                }
                frame 3 {
                  n670 = local write "100x gain"(w844) -> ()
                }
                frame 4, Default {
                }
              }
            }
          }
          frame #1 {
            n671 = local read "TEST STANDARD"() -> (w846:T3)
            n672 = case shown="\"ISO 12156\"" w846 {
              tunnel: ["ASTM D6079" "ISO 12156"] -> w845
              frame "ASTM D6079", Default {
              }
              frame "ISO 12156" {
              }
            }
            n673 = call "IMAGE ANALYSIS.vi"("Enum"=POST_ANALYSIS_ENUM."GET MEASUREMENTS", "error in"=w863) -> ("error out"=w870:errorcluster)  [unwired: 8 in, 1 out]
            n674 = local read "Magnification :"() -> (w856:string)
            n675 = call "Stall Data Flow.vim"("value in"=w870, "milliseconds to wait"=u32 1000) -> ("value out"=w869:errorcluster)  [unwired: 1 out]
            n676 = local read "Test File List :"() -> (w867:string)
            n677 = case shown="\"10x\"" w856 {
              tunnel: [w906 w907] -> w854
              frame "5x", Default {
                n678 = local read "5x Gain"() -> (w906:dbl)
              }
              frame "10x" {
                # "5x"
                n679 = local read "10x Gain"() -> (w907:dbl)
              }
            }
            n680 = call "IMAGE ANALYSIS.vi"("Enum"=POST_ANALYSIS_ENUM."READ", "error in"=w869) -> ("error out"=w866:errorcluster, "data out"=w857:string)  [unwired: 8 in]
            n681 = Match Pattern(string=w857, regular expression="\"type\": ") -> (after substring=w861:string)  [unwired: 1 in, 3 out]
            n682 = call "IMAGE PATH CREATION PY.vi"("error in (no error)"=w866, "File Name :"=w867) -> ("error out"=w865:errorcluster, "File Path"=w853:path, "File Path String:"=w848:string)  [unwired: 7 in]
            n683 = Match Pattern(string=w861, regular expression=",") -> (before substring=w847:string)  [unwired: 1 in, 3 out]
            n684 = local read "Calibration Tab"() -> (w850:enum32{"Measrument", "Calibrate"})
            n685 = call "Stall Data Flow.vim"("value in"=w865, "milliseconds to wait"=u32 250) -> ("value out"=w849:errorcluster)  [unwired: 1 out]
            n686 = Equal?(x=w847, y="\"rectangle\"") -> (x = y?=w858:bool)
            n687 = case shown="False" w858 {
              tunnel: w857 -> [w912 w967]
              tunnel: w854 -> [_ w958]
              tunnel: cluster{"major":dbl, "minor":dbl, "average":dbl} {"major"=0.0, "minor"=0.0, "average"=0.0} -> [w910 w954]
              tunnel: [w909 w951] -> w852
              tunnel: w847 -> [w911 _]
              tunnel: w854 -> [w908 _]
              frame False {
                n688 = Equal?(x=w911, y="\"line\"") -> (x = y?=w913:bool)
                n689 = case shown="True" w913 {
                  tunnel: w912 -> [_ w928]
                  tunnel: w910 -> [w915 w927]
                  tunnel: [w915 w925] -> w909
                  tunnel: w908 -> [_ w924]
                  frame False {
                  }
                  frame True {
                    w923 = 0.0 ("Major Axis")
                    n690 = Match Pattern(string=w928, regular expression="\"length_px\":") -> (after substring=w926:string)  [unwired: 1 in, 3 out]
                    n691 = property on="Major Axis" class="DigNum (strict)"("Caption.Text"="") -> ()  [unwired: 2 in, 2 out]
                    n692 = property on="Minor Axis" class="DigNum (strict)"("Caption.Text"="") -> ()  [unwired: 2 in, 2 out]
                    n693 = property on="Average" class="DigNum (strict)"("Caption.Text"="Line") -> ()  [unwired: 2 in, 2 out]
                    n694 = Fract/Exp String To Number(string=w926, default (0 dbl)=0.0 ("default (0 DBL)")) -> (number=w922:dbl)  [unwired: 2 in, 1 out]
                    "Pixel Value" <- w922
                    n695 = Multiply(x=w922, y=w924) -> (x*y=w935:dbl)
                    n696 = Multiply(x=w935, y=1000.0) -> (x*y=w918:dbl)
                    n697 = Divide(x=w918, y=1000.0) -> (x/y=w921:dbl)
                    n698 = local write "Measurment (mm)"(w921) -> ()
                    n699 = Bundle By Name(cluster=w927, "average"=w918) -> (w925:cluster{"major":dbl, "minor":dbl, "average":dbl})
                    n700 = Number To Fractional String(number=w918, precision (6)=i16 1) -> (F-format string=w917:string)  [unwired: 2 in]
                    n701 = local write "Minor Axis"(w923) -> ()
                    n702 = local write "Major Axis"(w923) -> ()
                    n703 = Fract/Exp String To Number(string=w917) -> (number=w916:dbl)  [unwired: 3 in, 1 out]
                    n704 = local write "Average"(w916) -> ()
                  }
                }
              }
              frame True {
                w955 = 1000.0 ("y")
                w961 = 0.0 ("default (0 DBL)")
                n705 = Match Pattern(string=w967, regular expression=" \"width_px\":") -> (after substring=w965:string)  [unwired: 1 in, 3 out]
                n706 = Match Pattern(string=w965, regular expression="\"height_px\":") -> (before substring=w963:string, after substring=w962:string)  [unwired: 1 in, 2 out]
                n707 = Fract/Exp String To Number(string=w963, default (0 dbl)=w961) -> (number=w960:dbl)  [unwired: 2 in, 1 out]
                n708 = Fract/Exp String To Number(string=w962, default (0 dbl)=w961) -> (number=w959:dbl)  [unwired: 2 in, 1 out]
                n709 = Multiply(x=w960, y=w958) -> (x*y=w957:dbl)
                n710 = Multiply(x=w959, y=w958) -> (x*y=w956:dbl)
                n711 = Multiply(x=w957, y=w955) -> (x*y=w941:dbl)
                n712 = Multiply(x=w956, y=w955) -> (x*y=w939:dbl)
                n713 = Add(x=w941, y=w939) -> (x+y=w953:dbl)
                n714 = property on="Major Axis" class="DigNum (strict)"("Caption.Text"="Major Axis") -> ()  [unwired: 2 in, 2 out]
                n715 = property on="Minor Axis" class="DigNum (strict)"("Caption.Text"="Minor Axis") -> ()  [unwired: 2 in, 2 out]
                n716 = property on="Average" class="DigNum (strict)"("Caption.Text"="Average") -> ()  [unwired: 2 in, 2 out]
                n717 = Divide(x=w953, y=2.0) -> (x/y=w937:dbl)
                n718 = Bundle By Name(cluster=w954, "major"=w941, "minor"=w939, "average"=w937) -> (w951:cluster{"major":dbl, "minor":dbl, "average":dbl})
                n719 = Number To Fractional String(number=w939, precision (6)=i16 1) -> (F-format string=w946:string)  [unwired: 2 in]
                n720 = Number To Fractional String(number=w937, precision (6)=i16 1) -> (F-format string=w947:string)  [unwired: 2 in]
                n721 = Number To Fractional String(number=w941, precision (6)=i16 1) -> (F-format string=w945:string)  [unwired: 2 in]
                n722 = Fract/Exp String To Number(string=w946) -> (number=w938:dbl)  [unwired: 3 in, 1 out]
                n723 = Fract/Exp String To Number(string=w947) -> (number=w936:dbl)  [unwired: 3 in, 1 out]
                n724 = Fract/Exp String To Number(string=w945) -> (number=w940:dbl)  [unwired: 3 in, 1 out]
                n725 = local write "Major Axis"(w940) -> ()
                n726 = local write "Average"(w936) -> ()
                n727 = local write "Minor Axis"(w938) -> ()
              }
            }
            n728 = case shown="\"Measrument\", Default" w850 {
              tunnel: w853 -> [w880 _]
              tunnel: w852 -> [w879 _]
              tunnel: [w876 w905] -> w851
              tunnel: w849 -> [w878 w905]
              tunnel: w848 -> [w877 _]
              tunnel: w845 -> [w875 _]
              frame "Measrument", Default {
                n729 = stacked-sequence {
                  tunnel: w880 -> [w898 _]
                  tunnel: w879 -> [w896 _]
                  tunnel: w878 -> [w894 _]
                  tunnel: w877 -> [w893 _]
                  tunnel: [w888 _] -> w876
                  tunnel: w875 -> [w881 _]
                  frame #0 {
                    n730 = call "IMAGE ANALYSIS.vi"("Enum"=POST_ANALYSIS_ENUM."SAVE IMAGE", "error in"=w894, "IMAGE FILE PATH"=w893) -> ("error out"=w892:errorcluster)  [unwired: 7 in, 1 out]
                    n731 = call "Stall Data Flow.vim"("value in"=w892, "milliseconds to wait"=u32 1000) -> ("value out"=w883:errorcluster)  [unwired: 1 out]
                    n732 = local read "Test File List :"() -> (w900:string)
                    n733 = call "IMAGE ANALYSIS.vi"("Enum"=POST_ANALYSIS_ENUM."MINIMIZE UI", "error in"=w883) -> ("error out"=w890:errorcluster)  [unwired: 8 in, 1 out]
                    n734 = Bundle By Name(cluster=T25 {"File Name"="", "Test Method"="", "Operator"="", "Fuel Description"="", "Date and time"=""} ("Main Ref"), "Test Method"=w881, "File Name"=w900) -> (w901:T25)
                    n735 = call "Stall Data Flow.vim"("value in"=w890, "milliseconds to wait"=u32 1500) -> ("value out"=w885:errorcluster)  [unwired: 1 out]
                    n736 = call "duf file read.vi"("error in (no error)"=w885, "Main Ref"=w901) -> ("error out"=w899:errorcluster, "Main Ref 2"=w897:T25)  [unwired: 8 in]
                    n737 = call "DETECTION REPORT for manual.vi"("error in (no error)"=w899, "return value 3"=w896, "Image File Path"=w898, "Main Ref"=w897) -> ("error out"=w895:errorcluster)  [unwired: 7 in]
                    n738 = call <vilib>:"Clear Errors.vi"("error in (no error)"=w895) -> ("error out"=w886:errorcluster)  [unwired: 5 in, 1 out]
                    n739 = call "IMAGE ANALYSIS.vi"("Enum"=POST_ANALYSIS_ENUM."MINIMIZE UI", "error in"=w886) -> ("error out"=w888:errorcluster)  [unwired: 8 in, 1 out]
                  }
                  frame #1 {
                    n740 = local write "Main Tab"(T2."HOME" ("Main Tab")) -> ()
                    n741 = local write "Main Dashboard Buttons"(T1."Home" ("Main Dashboard Buttons")) -> ()
                  }
                }
              }
              frame "Calibrate" {
              }
            }
          }
          frame #2 {
            n742 = Not(x=w970) -> (.not. x?=w969:bool)
            n743 = local write "Confirm Measrurement"(w969) -> ()
            n744 = local read "Calibration Tab"() -> (w968:enum32{"Measrument", "Calibrate"})
            n745 = case shown="\"Measrument\", Default" w968 {
              frame "Measrument", Default {
                (unwired) T20."HOME" ("Main Tab")
                n746 = local write "Main Tab"(T2."HOME" ("Main Tab")) -> ()
              }
              frame "Calibrate" {
              }
            }
          }
        }
      }
    }
    n747 = local read "Humidity"() -> (w713:bool)
    n748 = local read "Save Change"() -> (w718:bool)
    n749 = local read "Calibrate"() -> (w719:bool)
    n750 = local read "Auto Start Test"() -> (w714:bool)
    n751 = case shown="True" w719 {
      selector: w719 -> [_ w826]
      frame False {
      }
      frame True {
        n752 = Not(x=w826) -> (.not. x?=w825:bool)
        n753 = local write "Calibrate"(w825) -> ()
        n754 = local write "Calibration Tab"(enum32{"Measrument", "Calibrate"}."Calibrate" ("Calibration Tab")) -> ()
      }
    }
    n755 = case shown="True" w718 {
      selector: w718 -> [_ w770]
      frame False {
      }
      frame True {
        n756 = stacked-sequence {
          tunnel: w770 -> [_ _ _ _ w824]
          frame #0 {
            n757 = call "IMAGE ANALYSIS.vi"("Enum"=POST_ANALYSIS_ENUM."HIDE UI") -> ()  [unwired: 9 in, 2 out]
          }
          frame #1 {
            n758 = local read "100x gain"() -> (w772:dbl)
            n759 = local read "10x Gain"() -> (w773:dbl)
            n760 = local read "5x Gain"() -> (w774:dbl)
            n761 = Number To Fractional String(number=w773, width (-)=i16 4, precision (6)=i16 7) -> (F-format string=w795:string)  [unwired: 1 in]
            n762 = Number To Fractional String(number=0.0, width (-)=i16 4, precision (6)=i16 7) -> (F-format string=w790:string)  [unwired: 1 in]
            n763 = Number To Fractional String(number=w772, width (-)=i16 4, precision (6)=i16 7) -> (F-format string=w778:string)  [unwired: 1 in]
            n764 = Number To Fractional String(number=w774, width (-)=i16 10 ("precision (6)"), precision (6)=i16 7) -> (F-format string=w804:string)  [unwired: 1 in]
            n765 = Concatenate Strings("[CH1]" ("string"), w804, " - 5x Gain" ("string"), "\r") -> (w794:string)
            n766 = Concatenate Strings("[CH2]" ("string"), w795, " - 10x Gain" ("string"), "\r") -> (w793:string)
            n767 = Concatenate Strings("[CH3]" ("string"), w790, " - 20x Gain" ("string"), "\r") -> (w784:string)
            n768 = Concatenate Strings("[CH4]" ("string"), w778, " - 100x Gain" ("string"), "\r") -> (w777:string)
            n769 = String To Path(string="C:\\LAB-IQ\\Image Calibrate v01.dcf") -> (path=w807:path)
            n770 = Concatenate Strings(w794, w793, w784, w777) -> (w792:string)
            n771 = call <vilib>:"Write Characters To File.vi"("append to file? (new file:F)"=FALSE, "character string"=w792, "file path (dialog if empty)"=w807) -> ()  [unwired: 2 in, 1 out]
          }
          frame #2 {
            n772 = String To Path(string="C:\\LAB-IQ\\Image Calibrate v01.dcf") -> (path=w810:path)
            n773 = Open/Create/Replace File ("Open File")(file path (use dialog)=w810) -> (refnum out=w811:refnum<file>)  [unwired: 5 in, 2 out]
            n774 = for {
              N: 4 -> [_]
              tunnel: w811 -> [w817]
              i -> [w813]
              n775 = Read from Text File ("Read File")(file (use dialog)=w817) -> (text=w818:string)  [unwired: 3 in, 3 out]
              n776 = String Subset(string=w818, offset (0)=6, length (rest)=10 ("length (rest)")) -> (substring=w814:string)
              n777 = Fract/Exp String To Number(string=w814) -> (number=w812:dbl)  [unwired: 3 in, 1 out]
              n778 = case shown="3" w813 {
                tunnel: w812 -> [w819 w820 _ w821 _]
                frame 0 {
                  n779 = local write "5x Gain"(w819) -> ()
                }
                frame 1 {
                  n780 = local write "10x Gain"(w820) -> ()
                }
                frame 2 {
                }
                frame 3 {
                  n781 = local write "100x gain"(w821) -> ()
                }
                frame 4, Default {
                }
              }
            }
          }
          frame #3 {
            n782 = call "IMAGE ANALYSIS.vi"("Enum"=POST_ANALYSIS_ENUM."SHOW UI") -> ()  [unwired: 9 in, 2 out]
          }
          frame #4 {
            n783 = Not(x=w824) -> (.not. x?=w823:bool)
            n784 = local write "Save Change"(w823) -> ()
          }
        }
      }
    }
    n785 = case shown="False" w714 {
      tunnel: w713 -> [w740 _]
      frame False {
        n786 = case shown="True" w740 {
          frame False {
          }
          frame True {
            n787 = local read "Set Humidity:"() -> (w744:dbl)
            n788 = local read "Set Humidity:"() -> (w747:dbl)
            n789 = local read "Humidity ( %RH )"() -> (w748:dbl)
            n790 = Subtract(x=w744, y=2.0) -> (x-y=w742:dbl)
            n791 = Add(x=w747, y=2.0) -> (x+y=w743:dbl)
            n792 = In Range and Coerce(upper limit=w743, x=w748, lower limit=w742) -> (In Range?=w741:bool)  [unwired: 1 out]
            n793 = case shown="True" w741 {
              frame False {
              }
              frame True {
                n794 = case shown="True" "Manual Humididty Reached" {
                  selector: "Manual Humididty Reached" -> [_ w751]
                  frame False {
                  }
                  frame True {
                    n795 = Not(x=w751) -> (.not. x?=w750:bool)
                    n796 = local write "Manual Humididty Reached"(w750) -> ()
                    n797 = local read "EVENT LOG"() -> (w753:string)
                    n798 = call "Event Log.vi"("Content"="Target Humidity reached", "EVENT LOG"=w753) -> ("EVENT LOG"=w752:string)  [unwired: 8 in, 1 out]
                    n799 = local write "EVENT LOG"(w752) -> ()
                  }
                }
              }
            }
          }
        }
      }
      frame True {
        n800 = local write "Manual Humididty Reached"(TRUE ("Manual Humididty Reached")) -> ()
      }
    }
    n801 = local read "Cap Live Image"() -> (w734:bool)
    n802 = local read "SCAR MEASURMENT"() -> (w737:enum32{"Auto Scar", "Manual Scar"})
    n803 = Wait (ms)(milliseconds to wait=u32 250) -> ()  [unwired: 1 out]
    n804 = Equal?(x=w737, y=enum32{"Auto Scar", "Manual Scar"}."Manual Scar" ("SCAR MEASURMENT")) -> (x = y?=w735:bool)
    n805 = And(x=w735, y=w734) -> (x .and. y?=w733:bool)
    n806 = case shown="True" w733 {
      selector: w733 -> [_ w1049]
      frame False {
      }
      frame True {
        n807 = stacked-sequence {
          tunnel: [_ _ _ w1064 _] -> _
          tunnel: w1049 -> [_ _ _ _ w1071]
          frame #0 {
            w1050 = 0.0
            n808 = local write "Major Axis"(w1050) -> ()
            n809 = local write "Minor Axis"(w1050) -> ()
            n810 = local write "Average"(w1050) -> ()
          }
          frame #1 {
            n811 = call "CAMERA LIVE FEED FGV.vi"("Enum - Menu"=CAMERA_LIVE_FEED_ENUM."CAMERA MINIMIZE") -> ()  [unwired: 9 in, 2 out]
          }
          frame #2 {
            n812 = local read "FILE 3"() -> (w1058:string)
            n813 = call <vilib>:"Trim Whitespace.vi"("string"="C:\\LAB-IQ\\images\\") -> ("trimmed string"=w1060:string)  [unwired: 1 in]
            n814 = String To Path(string=w1060) -> (path=w1059:path)
            n815 = Concatenate Strings(w1058, ".png" ("string")) -> (w1057:string)
            n816 = Build Path(base path=w1059, name or relative path=w1057) -> (appended path=w1055:path)
            n817 = Path To String(path=w1055) -> (string=w1054:string)
            n818 = call "CAMERA LIVE FEED FGV.vi"("Enum - Menu"=CAMERA_LIVE_FEED_ENUM."CAMERA SAVE", "Image Path"=w1054) -> ("error out"=w1052:errorcluster)  [unwired: 8 in, 1 out]
            n819 = case shown="No Error" w1052 {
              frame No Error {
                n820 = One Button Dialog(message="Image saved successfully") -> ()  [unwired: 1 in, 1 out]
              }
              frame Error {
              }
            }
          }
          frame #3 {
            n821 = call "LIST FILE NAMES.vi"() -> ("error out"=w1066:errorcluster, "filenames"=w1063:string[])  [unwired: 10 in]
            n822 = call "IMAGE ANALYSIS.vi"("Enum"=POST_ANALYSIS_ENUM."SHOW UI", "error in"=w1066) -> ("error out"=w1064:errorcluster)  [unwired: 8 in, 1 out]
            n823 = property on="Test File List :" class="CmbBox"("Strings[]"=w1063) -> ()  [unwired: 2 in, 2 out]
          }
          frame #4 {
            (unwired) T24."Report" ("Main Dashboard Buttons")
            (unwired) T26."Report" ("Main Dashboard Buttons")
            n824 = Not(x=w1071) -> (.not. x?=w1070:bool)
            n825 = local write "Zoom Factore"(0.0 ("Zoom Factore")) -> ()
            n826 = local write "Cap Live Image"(w1070) -> ()
            n827 = local write "Main Tab"(T2."Adv Scar Report" ("Main Tab")) -> ()
            n828 = property on="Cap Live Image" class="Bool (strict)"("BoolText.Text"="Capture Image" ("Boolean Text.Text")) -> ()  [unwired: 2 in, 2 out]
            n829 = local write "Main Dashboard Buttons"(T1."Report" ("Main Dashboard Buttons")) -> ()
          }
        }
      }
    }
    n830 = local read "change Gain"() -> (w717:bool)
    n831 = local read "Back Square"() -> (w716:bool)
    n832 = case shown="True" w717 {
      selector: w717 -> [_ w761]
      frame False {
      }
      frame True {
        n833 = stacked-sequence {
          tunnel: w761 -> [_ w769]
          frame #0 {
            n834 = local read "Actual (µm)"() -> (w765:dbl)
            n835 = local read "Pixel Value"() -> (w764:dbl)
            n836 = local read "Magnification :"() -> (w763:string)
            n837 = Divide(x=w765, y=w764) -> (x/y=w762:dbl)
            n838 = case shown="\"10x\"" w763 {
              tunnel: w762 -> [w766 w767]
              frame "10x" {
                n839 = local write "10x Gain"(w766) -> ()
              }
              frame "5x", Default {
                n840 = local write "5x Gain"(w767) -> ()
              }
            }
          }
          frame #1 {
            n841 = Not(x=w769) -> (.not. x?=w768:bool)
            n842 = local write "change Gain"(w768) -> ()
          }
        }
      }
    }
    n843 = case shown="True" w716 {
      selector: w716 -> [_ w759]
      frame False {
      }
      frame True {
        n844 = Not(x=w759) -> (.not. x?=w758:bool)
        n845 = local write "Back Square"(w758) -> ()
        n846 = local write "Calibration Tab"(enum32{"Measrument", "Calibrate"}."Measrument" ("Calibration Tab")) -> ()
      }
    }
    n847 = local read "Rectangle Tool"() -> (w728:bool)
    n848 = local read "Clear ROI Tool"() -> (w727:bool)
    n849 = local read "Open Image"() -> (w732:bool)
    n850 = local read "line tool"() -> (w729:bool)
    n851 = local read "OUT"() -> (w730:bool)
    n852 = local read "In"() -> (w731:bool)
    n853 = case shown="True" w732 {
      selector: w732 -> [_ w1037]
      tunnel: [w1033 w1039] -> _
      tunnel: w722 -> [w1033 w1038]
      frame False {
      }
      frame True {
        n854 = Not(x=w1037) -> (.not. x?=w1036:bool)
        n855 = local write "Open Image"(w1036) -> ()
        n856 = call "IMAGE ANALYSIS.vi"("Enum"=POST_ANALYSIS_ENUM."HIDE UI", "error in"=w1038) -> ("error out"=w1046:errorcluster)  [unwired: 8 in, 1 out]
        n857 = call "File Dialog"("start path"=path "C:/LAB-IQ/images", "error in"=w1046) -> ("selected path"=w1035:path, "error out"=w1044:errorcluster)  [unwired: 10 in, 2 out]
        "Image path  2" <- w1035
        n858 = call <vilib>:"Clear Errors.vi"("error in (no error)"=w1044) -> ("error out"=w1043:errorcluster)  [unwired: 5 in, 1 out]
        n859 = call "IMAGE ANALYSIS.vi"("Enum"=POST_ANALYSIS_ENUM."OPEN FILE", "error in"=w1043, "File Path"=w1035) -> ("error out"=w1042:errorcluster)  [unwired: 7 in, 1 out]
        n860 = call <vilib>:"Clear Errors.vi"("error in (no error)"=w1042) -> ("error out"=w1041:errorcluster)  [unwired: 5 in, 1 out]
        n861 = call "IMAGE ANALYSIS.vi"("Enum"=POST_ANALYSIS_ENUM."SHOW UI", "error in"=w1041) -> ("error out"=w1039:errorcluster)  [unwired: 8 in, 1 out]
        n862 = local write "Zoom Factore"(100.0 ("Zoom Factore")) -> ()
      }
    }
    n863 = case shown="True" w730 {
      selector: w730 -> [_ w1018]
      tunnel: w722 -> [w1015 w1023]
      tunnel: [w1015 w1017] -> _
      frame False {
      }
      frame True {
        n864 = Not(x=w1018) -> (.not. x?=w1016:bool)
        n865 = local read "Zoom Factore"() -> (w1021:dbl)
        n866 = local write "OUT"(w1016) -> ()
        n867 = call "IMAGE ANALYSIS.vi"("Enum"=POST_ANALYSIS_ENUM."ZOOM OUT", "error in"=w1023) -> ("error out"=w1017:errorcluster)  [unwired: 8 in, 1 out]
        n868 = Divide(x=w1021, y=1.2) -> (x/y=w1019:dbl)
        n869 = local write "Zoom Factore"(w1019) -> ()
      }
    }
    n870 = case shown="True" w731 {
      selector: w731 -> [_ w1027]
      tunnel: w722 -> [w1024 w1032]
      tunnel: [w1024 w1025] -> _
      frame False {
      }
      frame True {
        n871 = Not(x=w1027) -> (.not. x?=w1026:bool)
        n872 = local read "Zoom Factore"() -> (w1030:dbl)
        n873 = local write "In"(w1026) -> ()
        n874 = call "IMAGE ANALYSIS.vi"("Enum"=POST_ANALYSIS_ENUM."ZOOM IN", "error in"=w1032) -> ("error out"=w1025:errorcluster)  [unwired: 8 in, 1 out]
        n875 = Multiply(x=w1030, y=1.2) -> (x*y=w1028:dbl)
        n876 = local write "Zoom Factore"(w1028) -> ()
      }
    }
    n877 = case shown="True" w727 {
      selector: w727 -> [_ w999]
      tunnel: w722 -> [w997 w1001]
      tunnel: [w997 w1000] -> _
      frame False {
      }
      frame True {
        n878 = Not(x=w999) -> (.not. x?=w998:bool)
        n879 = local write "Clear ROI Tool"(w998) -> ()
        n880 = call "IMAGE ANALYSIS.vi"("Enum"=POST_ANALYSIS_ENUM."CLEAR ROI", "error in"=w1001) -> ("error out"=w1000:errorcluster)  [unwired: 8 in, 1 out]
      }
    }
    n881 = case shown="True" w729 {
      selector: w729 -> [_ w1011]
      tunnel: w722 -> [w1009 w1014]
      tunnel: [w1009 w1012] -> _
      frame False {
      }
      frame True {
        n882 = Not(x=w1011) -> (.not. x?=w1010:bool)
        n883 = local write "line tool"(w1010) -> ()
        n884 = call "IMAGE ANALYSIS.vi"("Enum"=POST_ANALYSIS_ENUM."DRAW LINE", "error in"=w1014) -> ("error out"=w1012:errorcluster)  [unwired: 8 in, 1 out]
      }
    }
    n885 = case shown="True" w728 {
      selector: w728 -> [_ w1005]
      tunnel: w722 -> [w1003 w1007]
      tunnel: [w1003 w1006] -> _
      frame False {
      }
      frame True {
        n886 = Not(x=w1005) -> (.not. x?=w1004:bool)
        n887 = local write "Rectangle Tool"(w1004) -> ()
        n888 = call "IMAGE ANALYSIS.vi"("Enum"=POST_ANALYSIS_ENUM."DRAW REC", "error in"=w1007) -> ("error out"=w1006:errorcluster)  [unwired: 8 in, 1 out]
      }
    }
    n889 = local read "SCAR MEASURMENT"() -> (w715:enum32{"Auto Scar", "Manual Scar"})
    n890 = local read "Fit to Screen Tool"() -> (w724:bool)
    n891 = local read "Resize Tool"() -> (w723:bool)
    n892 = case shown="\"Manual Scar\", Default" w715 {
      frame "Auto Scar" {
        n893 = property on="Cap Live Image" class="Bool (strict)"("BoolText.Text"="Report" ("Boolean Text.Text")) -> ()  [unwired: 2 in, 2 out]
      }
      frame "Manual Scar", Default {
        n894 = property on="Cap Live Image" class="Bool (strict)"("BoolText.Text"="Save Image" ("Boolean Text.Text")) -> ()  [unwired: 2 in, 2 out]
      }
    }
    n895 = local read "ROI Color Tool"() -> (w725:bool)
    n896 = local read "Pan Tool"() -> (w726:bool)
    n897 = case shown="True" w726 {
      selector: w726 -> [_ w993]
      tunnel: w722 -> [w991 w995]
      tunnel: [w991 w994] -> _
      frame False {
      }
      frame True {
        n898 = Not(x=w993) -> (.not. x?=w992:bool)
        n899 = call "IMAGE ANALYSIS.vi"("Enum"=POST_ANALYSIS_ENUM."PAN", "error in"=w995) -> ("error out"=w994:errorcluster)  [unwired: 8 in, 1 out]
        n900 = local write "Pan Tool"(w992) -> ()
      }
    }
    n901 = case shown="True" w723 {
      selector: w723 -> [_ w977]
      tunnel: w722 -> [w972 w974]
      tunnel: [w972 w973] -> _
      frame False {
      }
      frame True {
        n902 = Not(x=w977) -> (.not. x?=w976:bool)
        n903 = local write "Resize Tool"(w976) -> ()
        n904 = call "IMAGE ANALYSIS.vi"("Enum"=POST_ANALYSIS_ENUM."RESIZE MODE", "error in"=w974) -> ("error out"=w973:errorcluster)  [unwired: 8 in, 1 out]
      }
    }
    n905 = case shown="True" w724 {
      selector: w724 -> [_ w982]
      tunnel: [w978 w983] -> _
      tunnel: w722 -> [w978 w981]
      frame False {
      }
      frame True {
        n906 = Not(x=w982) -> (.not. x?=w980:bool)
        n907 = local write "Zoom Factore"(100.0 ("Zoom Factore")) -> ()
        n908 = local write "Fit to Screen Tool"(w980) -> ()
        n909 = call "IMAGE ANALYSIS.vi"("Enum"=POST_ANALYSIS_ENUM."FIT", "error in"=w981) -> ("error out"=w983:errorcluster)  [unwired: 8 in, 1 out]
      }
    }
    n910 = case shown="True" w725 {
